vi "RolloverContinued.vi"(7 "acq block size (s)":dbl=1.0, 8 "rollover state":T1, 10 "OSClkStart":dbl, 11 "counter":u32[](array[numeric])) -> (0 "rollover state":T1, 2 "next block":dbl[](array[numeric]), 3 "this block":dbl[](array[numeric]), 5 "rolled over":bool)   [LabVIEW 2017]
uses:
  <vilib>/addons/InsightCM/Utilities/Misc/rolloverState.ctl
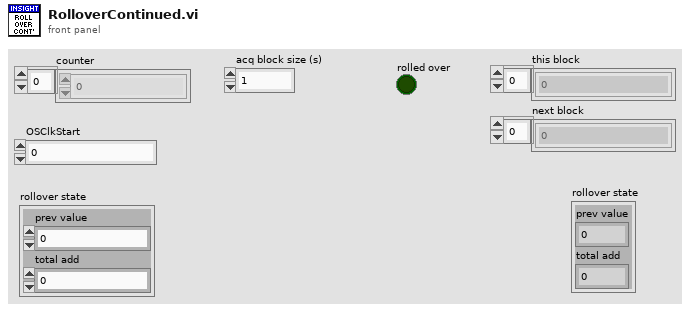
[diagram p1: front panel]
types:
  T1 = typedef "rolloverState.ctl" = cluster{"prev value":u32, "total add":dbl}
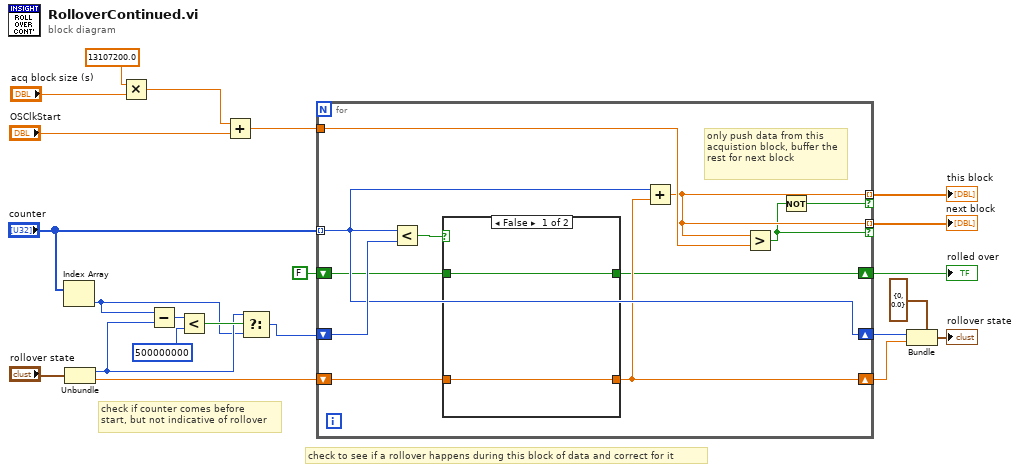
[diagram p0: block diagram]
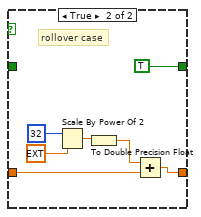
[diagram p2: hidden frame]
diagram:
  # "check if counter comes before\nstart, but not indicative of rollover"
  # "check to see if a rollover happens during this block of data and correct for it"
  n1 = Index Array(array="counter") -> (element=w2:u32)  [unwired: 1 in]
  n2 = Unbundle("rollover state") -> ("prev value"=w3:u32, "total add"=w5:dbl)
  n3 = Multiply(x=13107200.0, y="acq block size (s)") -> (x*y=w12:dbl)
  n4 = Subtract(x=w2, y=w3) -> (x-y=w7:u32)
  n5 = Less?(x=w7, y=u32 500000000) -> (x < y?=w4:bool)
  n6 = Add(x=w12, y="OSClkStart") -> (x+y=w15:dbl)
  n7 = Select(t=w3, s=w4, f=w2) -> (s? t:f=w1:u32)
  n8 = for {
    tunnel: "counter" -> [w30] mode=indexing
    shift-right: [w30] -> w21
    shift-left: w1 -> [w33]
    shift-right: [w29] -> w20
    shift-left: w5 -> [w31]
    tunnel: [w27] -> w22 mode=indexing if=w26
    tunnel: w15 -> [w28]
    tunnel: [w27] -> w14 mode=indexing if=w25
    shift-right: [w24] -> w9
    shift-left: FALSE -> [w23]
    # "only push data from this acquistion block, buffer the rest for next block"
    n9 = Less?(x=w30, y=w33) -> (x < y?=w32:bool)
    n10 = case shown="False" w32 {
      tunnel: w31 -> [w35 w42]
      tunnel: [w35 w39] -> w29
      tunnel: [w34 TRUE] -> w24
      tunnel: w23 -> [w34 _]
      frame False {
      }
      frame True {
        # "rollover case"
        n11 = Scale By Power Of 2(n=i16 32, x=ext 1.0) -> (x*2^n=w38:ext)
        n12 = To Double Precision Float(number=w38) -> (double precision float=w37:dbl)
        n13 = Add(x=w37, y=w42) -> (x+y=w39:dbl)
      }
    }
    n14 = Add(x=w30, y=w29) -> (x+y=w27:dbl)
    n15 = Greater?(x=w27, y=w28) -> (0:w25:bool)
    n16 = Not(x=w25) -> (.not. x?=w26:bool)
  }
  "this block" <- w22
  "next block" <- w14
  "rolled over" <- w9
  n17 = Bundle(cluster=T1 {"prev value"=0, "total add"=0.0}, "prev value"=w21, "total add"=w20) -> (→"rollover state":T1)
